vi "Sub Initialize.vi"(8 "error in (no error)":errorcluster, 11 "Channel Scanner in":refnum<class "Channel Scanner.lvclass">) -> (0 "error out":errorcluster, 2 "Initialize Result":refnum<class "Acquired Result.lvclass">, 3 "Channel Scanner out":refnum<class "Channel Scanner.lvclass">)   [LabVIEW 2019, in "Channel Scanner.lvclass"]
uses:
  Channel Scanner.lvclass
  C:/Program Files/National Instruments/LabVIEW 2019/vi.lib/ActorFramework/Actor/Actor.lvclass
  NHMFL_Core/Libraries/Instruments/Results/Acquired Result/Acquired Result.lvclass
  NHMFL_Core/Libraries/Instruments/Instrument Driver/Channel Scanner Driver/Channel Scanner Driver.lvclass/Channel Scanner Driver.ctl
  <vilib>/ActorFramework/Actor/Actor.lvclass/Actor.ctl
  <vilib>/ActorFramework/Message Enqueuer/Message Enqueuer.lvclass/Message Enqueuer.ctl
  Template Module Messages/Subscribe Request Msg/Subscribe Request Msg.lvclass/Subscribe Request Msg.ctl
  Channel Scanner.lvclass/Channel Scanner.ctl
  NHMFL_Core/Libraries/Instruments/Instrument Driver/Channel Scanner Driver/Write Next channel idx.vi
  NHMFL_Core/Libraries/Instruments/Instrument Driver/Channel Scanner Driver/Write Scan Channels.vi
  <vilib>/ActorFramework/Message Enqueuer/Init from Existing Queue.vi
  <vilib>/ActorFramework/Message Enqueuer/Enqueue.vi
  Template Module Messages/Subscribe Request Msg/Subscribe Request Msg.lvclass
  C:/Program Files/National Instruments/LabVIEW 2019/vi.lib/ActorFramework/Message/Message.lvclass
  Read Scanner driver.vi
  Read Channel scanner configuration.vi
  Write Scanner driver.vi
  <vilib>/ActorFramework/Message Priority Queue/Priority Enqueue.vi
  NHMFL_Core/Libraries/Instruments/Instrument Driver/Channel Scanner Driver/Channel Scanner Driver.lvclass
  <vilib>/ActorFramework/Message Enqueuer/Message Enqueuer.lvclass
  Instrument Actor/Instrument Actor.lvclass
  <vilib>/ActorFramework/Actor/Actor.lvclass
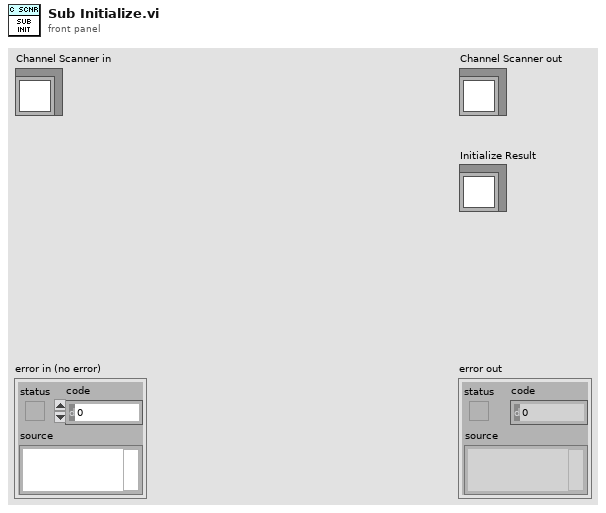
[diagram p1: front panel]
types:
  T1 = typedef "Channel Scanner Configuration.ctl" = cluster{"Scan channels":i32[], "Group with measurement":string}
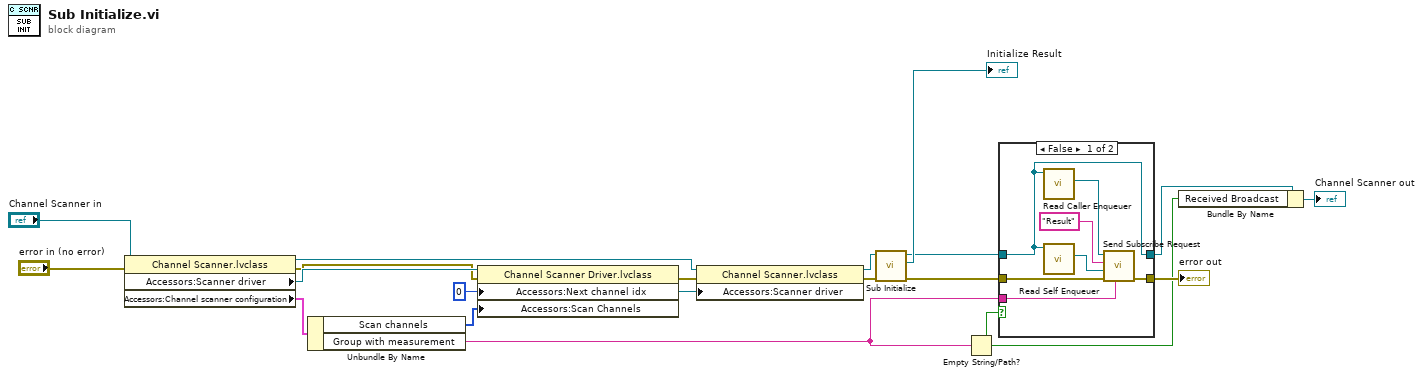
[diagram p0: block diagram]
diagram:
  n1 = property class="Channel Scanner.lvclass"(reference="Channel Scanner in", error in="error in (no error)") -> (reference out=w12:refnum<class "Channel Scanner.lvclass">, error out=w1:errorcluster, "Accessors:Scanner driver"=w18:refnum<class "Channel Scanner Driver.lvclass">, "Accessors:Channel scanner configuration"=w16:T1)
  n2 = Unbundle By Name(w16) -> ("Scan channels"=w15:i32[], "Group with measurement"=w8:string)
  n3 = property class="Channel Scanner Driver.lvclass"(reference=w18, error in=w1, "Accessors:Next channel idx"=0 ("Next channel idx"), "Accessors:Scan Channels"=w15) -> (reference out=w13:refnum<class "Channel Scanner Driver.lvclass">, error out=w14:errorcluster)
  n4 = property class="Channel Scanner.lvclass"(reference=w12, error in=w14, "Accessors:Scanner driver"=w13) -> (reference out=w10:refnum<class "Channel Scanner.lvclass">, error out=w11:errorcluster)
  n5 = call-parent "Sub Initialize.vi"("error in (no error)"=w11, "Instrument Recorder in"=w10) -> ("error out"=w5:errorcluster, "Initialize Result"=→"Initialize Result":refnum<class "Acquired Result.lvclass">, "Instrument Recorder out"=w7:refnum<class "Channel Scanner.lvclass">)  [unwired: 7 in]
  n6 = Empty String/Path?(string/path=w8) -> (empty?=w2:bool)
  n7 = case shown="False" w2 {
    tunnel: w8 -> [w25 _]
    tunnel: w7 -> [w22 w29]
    tunnel: [w22 w29] -> w6
    tunnel: w5 -> [w27 w28]
    tunnel: [w26 w28] -> w4
    frame False {
      n8 = call <vilib>:"Read Caller Enqueuer.vi"("Actor"=w22) -> ("Caller Enqueuer"=w23:refnum<class "Message Enqueuer.lvclass">)  [unwired: 10 in]
      n9 = call <vilib>:"Read Self Enqueuer.vi"("Actor"=w22) -> ("Self Enqueuer"=w21:refnum<class "Message Enqueuer.lvclass">)  [unwired: 10 in]
      n10 = call "Send Subscribe Request.vi"("Broadcaster"=w25, "error in (no error)"=w27, "Subscriber Enqueuer"=w21, "Topic"="Result", "Message Enqueuer"=w23) -> ("error out"=w26:errorcluster)  [unwired: 5 in, 1 out]
    }
    frame True {
    }
  }
  "error out" <- w4
  n11 = Bundle By Name(cluster=w6, "Received Broadcast"=w2) -> (→"Channel Scanner out":refnum<class "Channel Scanner.lvclass">)
